vi "XYZTheta-2Zspeed Go.vi"(8 "error in (no error)":errorcluster, 10 "XYZTheta In":dbl[](array[numeric]), 11 "Motion in":refnum<class "Motion.lvclass">) -> (0 "error out":errorcluster, 3 "Motion out":refnum<class "Motion.lvclass">)   [LabVIEW 2016, in "Motion.lvclass"]
uses:
  Motion.lvclass
panel:
  out "XYZTheta Out":dbl[](array[numeric])
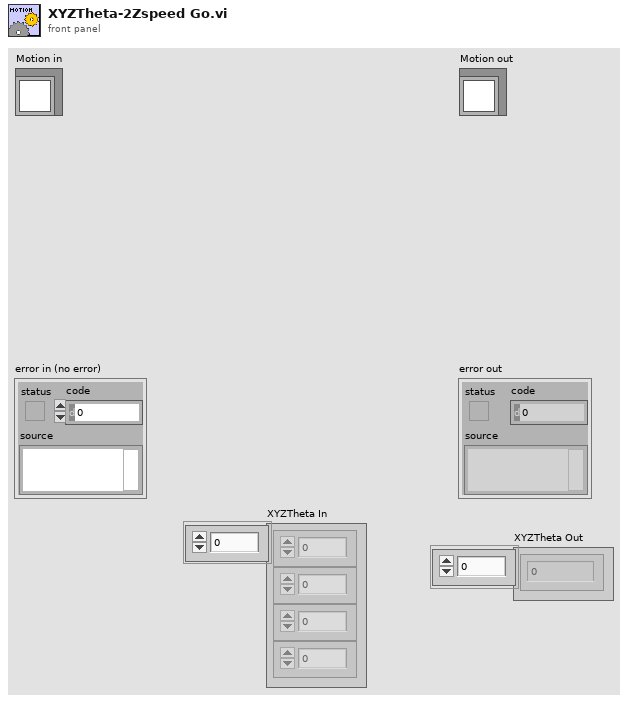
[diagram p1: front panel]
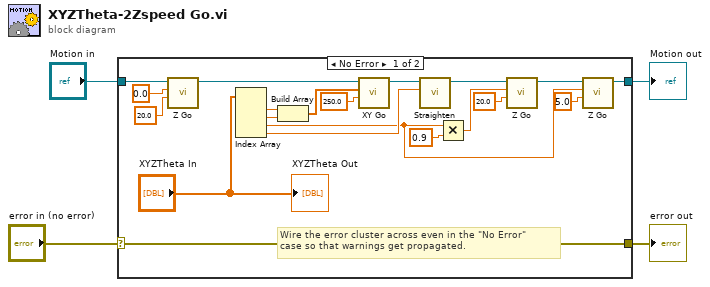
[diagram p0: block diagram]
diagram:
  n1 = case shown="No Error" "error in (no error)" {
    selector: "error in (no error)" -> [w24 w26]
    tunnel: [w24 w26] -> w3
    tunnel: [w13 w25] -> w1
    tunnel: "Motion in" -> [w6 w25]
    frame No Error {
      # "Wire the error cluster across even in the \"No Error\"\ncase so that warnings get propagated."
      n2 = call-dynamic "Z Go.vi"("Speed"=20.0, "Position"=0.0, "Motion in"=w6) -> ("Motion out"=w5:refnum<class "Motion.lvclass">)  [unwired: 7 in, 1 out]
      n3 = Index Array(array="XYZTheta In") -> (element #1=w21:dbl, element #2=w22:dbl, element #3=w9:dbl, element #4=w23:dbl)  [unwired: 4 in]
      n4 = Build Array(w21, w22) -> (w20:dbl[])
      n5 = call-dynamic "XY Go.vi"("Speed"=250.0, "XY"=w20, "Motion in"=w5) -> ("Motion out"=w18:refnum<class "Motion.lvclass">)  [unwired: 7 in, 1 out]
      n6 = call-dynamic "Straighten.vi"("Theta"=w23, "Motion in"=w18) -> ("Motion out"=w17:refnum<class "Motion.lvclass">)  [unwired: 8 in, 1 out]
      n7 = Multiply(x=w9, y=0.9) -> (x*y=w11:dbl)
      n8 = call-dynamic "Z Go.vi"("Speed"=20.0, "Position"=w11, "Motion in"=w17) -> ("Motion out"=w14:refnum<class "Motion.lvclass">)  [unwired: 7 in, 1 out]
      n9 = call-dynamic "Z Go.vi"("Speed"=5.0, "Position"=w9, "Motion in"=w14) -> ("Motion out"=w13:refnum<class "Motion.lvclass">)  [unwired: 7 in, 1 out]
      "XYZTheta Out" <- "XYZTheta In"
    }
    frame Error {
    }
  }
  "error out" <- w3
  "Motion out" <- w1
